vi "ChangeautoODs.vi"() -> ()   [LabVIEW 2015]
panel:
  in  "point OD":u16(ring)=4 items=["OD 0"=1, "OD 0.5"=2, "OD 1"=3, "OD 2"=4, "OD 3"=5, "OD 4"=6]
  in  "contour OD":u16(ring)=3 items=["OD 0"=1, "OD 0.5"=2, "OD 1"=3, "OD 2"=4, "OD 3"=5, "OD 4"=6]
  in  "image OD":u16(ring)=1 caption="Image OD" items=["OD 0"=1, "OD 0.5"=2, "OD 1"=3, "OD 2"=4, "OD 3"=5, "OD 4"=6]
  in  "OK Button":bool
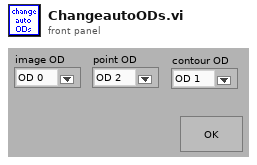
[diagram p1: front panel]
types:
  T1 = cluster{"StageS":i32, "StageL":i32, "currmeas data dir":path, "image OD":u16, "contour OD":u16, "point OD":u16, "AOlines":tag[], "AIlines":tag[], "CI lines":tag[], "DO lines":tag[], "AO names":string[], "CI names":string[], "AI names":string[], "DO names":string[], "CIextensions":string[], "AIextensions":string[], "Voltage to Ygalvo":i32, "Voltage to Xgalvo":i32, "Voltage to patch":i32, "640 shutter":i32, "2P shutter":i32, "LT timestamp":u32, "Vp":i32, "Ip":i32, "camera trigger":i32, "master data dir":path, "voltage to Zpos":i32, "Vto2P":i32, "640 AO":i32, "488 AO":i32, "532 AO":i32, "640TTL":u32, "488TTL":u32, "532TTL":u32, "Device 1 sampleclock out":tag, "Device 1 Starttrigger out":tag, "Device 2 sampleclock in":tag, "Device 2 StartTrigger in ":tag}
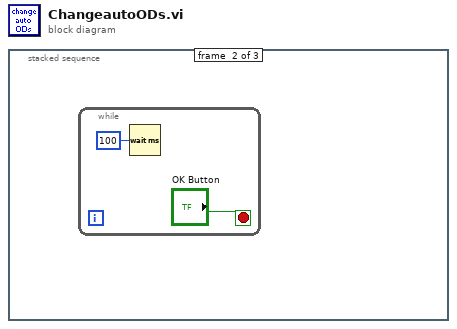
[diagram p0: block diagram]
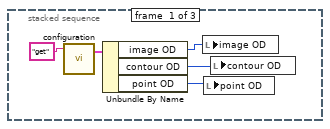
[diagram p2: hidden frame]
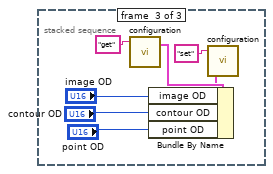
[diagram p3: hidden frame]
diagram:
  n1 = stacked-sequence {
    frame #0 {
      n2 = call "configuration.vi"("command"="get") -> ("config out"=w4:T1)  [unwired: 2 in, 1 out]
      n3 = Unbundle By Name(w4) -> ("image OD"=w1:u16, "contour OD"=w3:u16, "point OD"=w2:u16)
      n4 = local write "image OD"(w1) -> ()
      n5 = local write "point OD"(w2) -> ()
      n6 = local write "contour OD"(w3) -> ()
    }
    frame #1 {
      n7 = while {
        stop <- "OK Button" stop-if-true
        n8 = Wait (ms)(milliseconds to wait=u32 100) -> ()  [unwired: 1 out]
      }
    }
    frame #2 {
      n9 = call "configuration.vi"("command"="get") -> ("config out"=w12:T1)  [unwired: 2 in, 1 out]
      n10 = Bundle By Name(cluster=w12, "image OD"="image OD", "contour OD"="contour OD", "point OD"="point OD") -> (w11:T1)
      n11 = call "configuration.vi"("config in"=w11, "command"="set") -> ()  [unwired: 1 in, 2 out]
    }
  }
